vi "Channel Selection Dialog.vi"(8 "error in (no error)":errorcluster, 9 "NIVS.System Definition Root":refnum<k24>, 10 "NodePath":string, 11 "NodePathArray":string[](array[string])) -> (0 "error out":errorcluster, 2 "Selected NodePath":string, 3 "Selected NodePathArray":string[](array[string]))   [LabVIEW 2010]
doc: "Use this template to create a dialog box with event handling."
uses:
  NationalInstruments.VeriStand.SystemStorageUI
  NationalInstruments.VeriStand.SystemStorage
  <vilib>/NI Veristand/UI Controls/Single Node Browser/NI_VS UI Single Node Browser.lvlib
panel:
  in  "Cancel":bool
  in  "Ok":bool
  in  "Selected Channel":refnum<k24>(container)
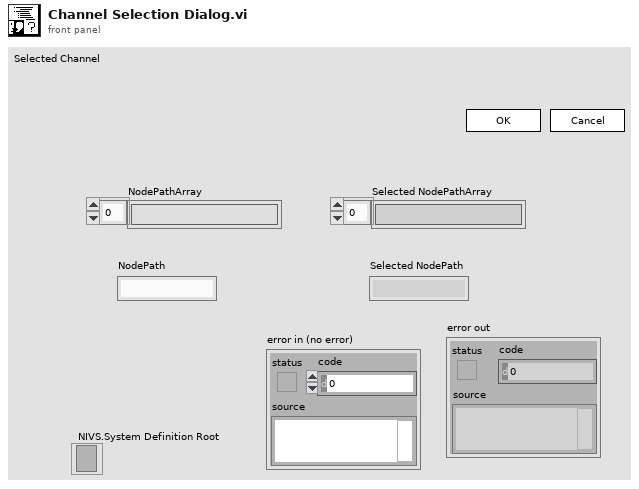
[diagram p1: front panel]
types:
  T1 = typedef "NI_VS UI Single Node Browser.lvlib/Callback Type.ctl" = cluster{"Net Callbacks":refnum<k27>[], "Event":refnum<user-event>}
  T2 = typedef "NI_VS UI Single Node Browser.lvlib/Node Ref.ctl" = refnum<k24>
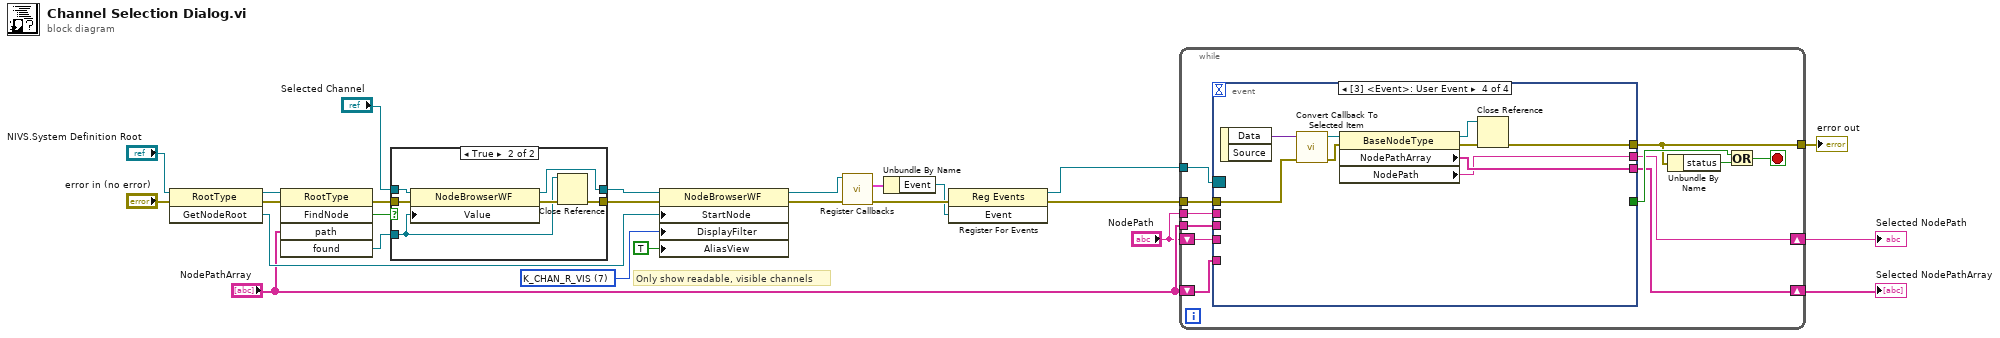
[diagram p0: block diagram]
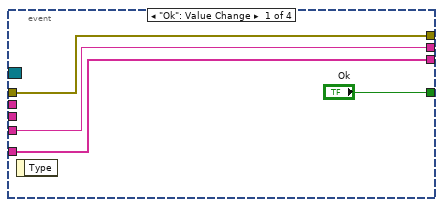
[diagram p3: hidden frame]
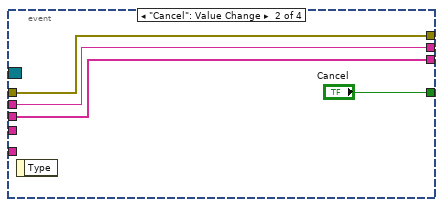
[diagram p4: hidden frame]
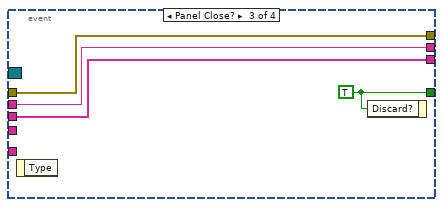
[diagram p5: hidden frame]
diagram:
  w14 = u8 7 items=["K_CHAN_R", "K_CHAN_W", "K_CHAN_RW", "K_CHAN_VOLT", "K_CHAN_FAULT", "K_ALL", "K_CUSTOM", "K_CHAN_R_VIS", "K_CHAN_W_VIS", "K_CHAN_RW_VIS", "K_CHAN_VOLT_VIS", "K_CHAN_FAULT_VIS"] ("DisplayFilter")
  # "Only show readable, visible channels"
  n1 = invoke class="RootType" method="GetNodeRoot"(reference="NIVS.System Definition Root", error in="error in (no error)") -> (reference out=w19:refnum<k24>, error out=w20:errorcluster, "GetNodeRoot"=w18:refnum<k24>)  [unwired: 1 in]
  n2 = invoke class="RootType" method="FindNode"(reference=w19, error in=w20, "path"="NodePathArray") -> (error out=w11:errorcluster, "FindNode"=w9:bool, "found"=w12:refnum<k24>)  [unwired: 2 in, 2 out]
  n3 = case shown="True" w9 {
    tunnel: w12 -> [_ w28]
    tunnel: w11 -> [w27 w29]
    tunnel: [w27 w32] -> w10
    tunnel: "Selected Channel" -> [w26 w31]
    tunnel: [w26 w30] -> w8
    frame False {
    }
    frame True {
      n4 = property class="NodeBrowserWF"(reference=w31, error in=w29, "Value"=w28) -> (reference out=w30:refnum<k24>, error out=w33:errorcluster)
      n5 = Close Reference(reference=w28, error in (no error)=w33) -> (error out=w32:errorcluster)
    }
  }
  n6 = property class="NodeBrowserWF"(reference=w8, error in=w10, "StartNode"=w18, "DisplayFilter"=w14, "AliasView"=TRUE) -> (reference out=w15:refnum<k24>, error out=w16:errorcluster)
  n7 = call <vilib>:"Register Callbacks.vi"("error in (no error)"=w16, "Single Node Browser"=w15) -> ("error out"=w24:errorcluster, "Callbacks"=w17:T1)  [unwired: 7 in, 1 out]
  n8 = Unbundle By Name(w17) -> ("Event"=w6:refnum<user-event>)
  n9 = register-events(error in=w24, w6) -> (reference out=w23:refnum<event-registration>, error out=w1:errorcluster)  [unwired: 1 in]
  n10 = while {
    tunnel: [w43] -> w25
    tunnel: w1 -> [w44]
    tunnel: w23 -> [w40]
    shift-right: [w39] -> w5
    shift-left: "NodePathArray" -> [w38]
    tunnel: "NodePathArray" -> [w37]
    shift-right: [w36] -> w3
    shift-left: "NodePath" -> [w35]
    tunnel: "NodePath" -> [w34]
    stop <- w42 stop-if-true
    n11 = event shown="[3] <Event>: User Event" {
      selector: w40 -> [_ _ _ _]
      dyn-events: _ -> [_ _ _ _]
      timeout: _ -> [_ _ _ _]
      tunnel: ["Ok" "Cancel" w57 _] -> w45
      tunnel: [w49 w52 w56 w64] -> w43
      tunnel: w44 -> [w49 w52 w56 w65]
      tunnel: [w47 w51 w55 w59] -> w39
      tunnel: w38 -> [w47 _ _ _]
      tunnel: w37 -> [_ w51 w55 _]
      tunnel: [w46 w50 w54 w58] -> w36
      tunnel: w35 -> [w46 _ _ _]
      tunnel: w34 -> [_ w50 w54 _]
      event "Ok": Value Change {
        n12 = event-data() -> ()  [unwired: 1 in, 1 out]
      }
      event "Cancel": Value Change {
        n13 = event-data() -> ()  [unwired: 1 in, 1 out]
      }
      event Panel Close? {
        w57 = TRUE ("Cancel")
        n14 = event-data() -> ()  [unwired: 1 in, 1 out]
        n15 = event-data("Discard?"=w57) -> ()  [unwired: 1 in, 1 out]
      }
      event User Event {
        n16 = event-data() -> ("Data"=w66:variant)  [unwired: 1 in, 1 out]
        n17 = call <vilib>:"Convert Callback To Selected Item.vi"("error in"=w65, "Data"=w66) -> ("error out"=w60:errorcluster, "Selected Item"=w63:T2)  [unwired: 8 in]
        n18 = property class="BaseNodeType"(reference=w63, error in=w60) -> (reference out=w62:T2, error out=w61:errorcluster, "NodePathArray"=w59:string[], "NodePath"=w58:string)
        n19 = Close Reference(reference=w62, error in (no error)=w61) -> (error out=w64:errorcluster)
      }
    }
    n20 = Unbundle By Name(w43) -> ("status"=w41:bool)
    n21 = Or(x=w45, y=w41) -> (x .or. y?=w42:bool)
  }
  "error out" <- w25
  "Selected NodePathArray" <- w5
  "Selected NodePath" <- w3
